vi "Display Data Queue manager.vi"(5 "queue size":i32, 7 "Action":T1=enum."Enqueue", 8 "error in":errorcluster, 11 "Data in":sgl[](array[numeric])) -> (0 "error out":errorcluster, 1 "# elements in queue":i32, 2 "Empty?":bool, 3 "data out":sgl[](array[numeric]))   [LabVIEW 2018]
uses:
  Controls/Queue Manager Actions.ctl
  Controls/QueueNames.ctl
  Controls/MessagePacket.ctl
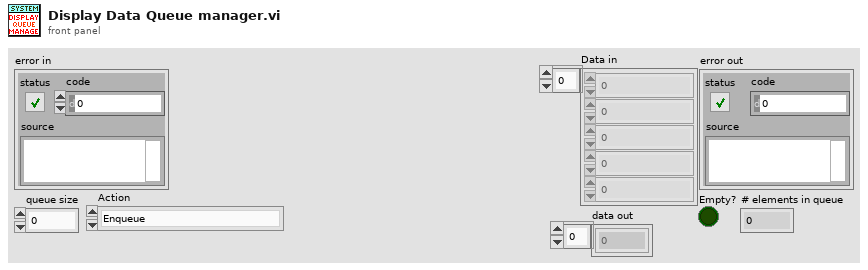
[diagram p1: front panel]
types:
  T1 = typedef "Queue Manager Actions.ctl" = enum16{"Init", "Enqueue", "Enqueue All", "Preview Queue", "Dequeue", "Get Status", "Flush Queue", "Flush All Queues", "Release All Queues", "Release Queue", "Enqueue at Opposite End"}
  T2 = typedef "MessagePacket.ctl" = cluster{"Message":string, "Parameter":variant}
  T3 = typedef "QueueNames.ctl" = enum16{"Main GUI", "Main Scan Processor", "Main Display Processing", "Main Processing", "Main Saving", "Main Display", "Main Table Stage GUI", "Main Table Stage Proc.", "Scan Engine", "Vibratome GUI", "Vibratome Processor", "Slice Engine"}
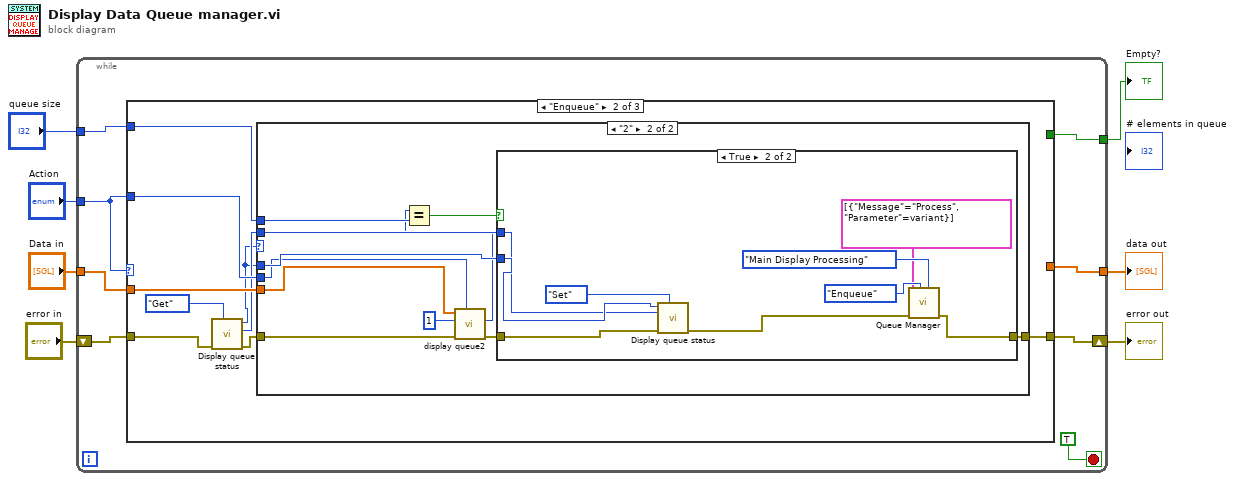
[diagram p0: block diagram]
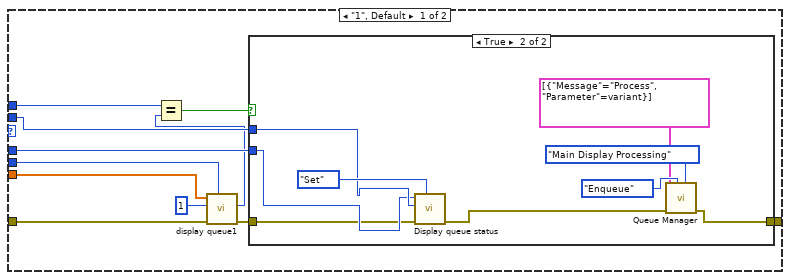
[diagram p3: hidden frame]
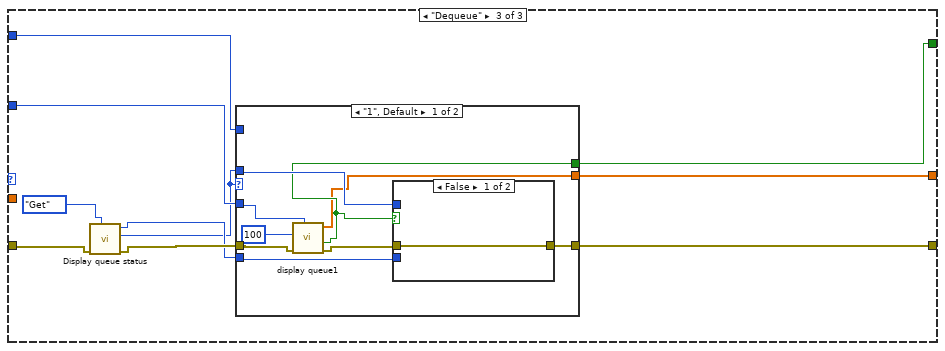
[diagram p6: hidden frame]
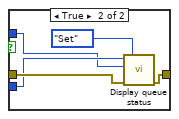
[diagram p7: hidden frame]
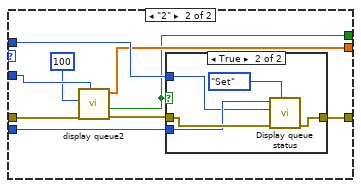
[diagram p8: hidden frame]
diagram:
  n1 = while {
    tunnel: "Data in" -> [w15]
    tunnel: "Action" -> [w14]
    tunnel: "queue size" -> [w12]
    shift-right: [w11] -> w3
    shift-left: "error in" -> [w13]
    tunnel: [w9] -> w2
    tunnel: [w8] -> w1
    stop <- TRUE stop-if-true
    n2 = case shown="\"Enqueue\"" w14 {
      tunnel: w15 -> [_ w25 _]
      tunnel: w13 -> [w16 w21 w72]
      tunnel: w14 -> [_ w24 w77]
      tunnel: w12 -> [_ w23 w76]
      tunnel: [w16 w22 w75] -> w11
      tunnel: [_ _ w74] -> w9
      tunnel: [_ _ w73] -> w8
      frame "Init", Default {
      }
      frame "Enqueue" {
        n3 = call "Display queue status.vi"("action"=enum16{"Init", "Get", "Set"}."Get", "error in"=w21) -> ("error out"=w17:errorcluster, "dequeue channel out"=w19:enum16{"1", "2"}, "enqueue channel out"=w18:enum16{"1", "2"})  [unwired: 6 in]
        n4 = case shown="\"2\"" w18 {
          tunnel: w25 -> [w31 w49]
          tunnel: w24 -> [w28 w51]
          tunnel: w17 -> [w27 w48]
          tunnel: w23 -> [w35 w57]
          tunnel: w18 -> [w33 w55]
          tunnel: w19 -> [w34 w54]
          tunnel: [w32 w53] -> w22
          frame "1", Default {
            n5 = call "display queue1.vi"("Action"=w28, "error in (no error)"=w27, "timeout in ms (-1)"=1, "data in"=w31) -> ("error out"=w29:errorcluster, "# elements in queue"=w26:i32)  [unwired: 4 in, 2 out]
            n6 = Equal?(x=w35, y=w26) -> (x = y?=w36:bool)
            n7 = case shown="True" w36 {
              tunnel: [w37 w40] -> w32
              tunnel: w29 -> [w37 w38]
              tunnel: w34 -> [_ w45]
              tunnel: w33 -> [_ w44]
              frame False {
              }
              frame True {
                n8 = call "Display queue status.vi"("action"=enum16{"Init", "Get", "Set"}."Set", "error in"=w38, "enqueue channel in"=w45, "dequeue channel in"=w44) -> ("error out"=w39:errorcluster)  [unwired: 4 in, 2 out]
                n9 = call "Queue Manager.vi"("Queue Name"=QueueNames."Main Display Processing", "Action"=Queue_Manager_Actions."Enqueue", "Error In"=w39, "Message Packet Array"=T2[] [{"Message"="Process", "Parameter"=variant}]) -> ("Error Out"=w40:errorcluster)  [unwired: 3 in, 4 out]
              }
            }
          }
          frame "2" {
            n10 = call "display queue2.vi"("Action"=w51, "error in (no error)"=w48, "timeout in ms (-1)"=1, "data in"=w49) -> ("error out"=w52:errorcluster, "# elements in queue"=w47:i32)  [unwired: 4 in, 2 out]
            n11 = Equal?(x=w47, y=w57) -> (x = y?=w56:bool)
            n12 = case shown="True" w56 {
              tunnel: w52 -> [w58 w60]
              tunnel: w55 -> [_ w66]
              tunnel: w54 -> [_ w65]
              tunnel: [w58 w61] -> w53
              frame False {
              }
              frame True {
                n13 = call "Display queue status.vi"("action"=enum16{"Init", "Get", "Set"}."Set", "error in"=w60, "enqueue channel in"=w65, "dequeue channel in"=w66) -> ("error out"=w59:errorcluster)  [unwired: 4 in, 2 out]
                n14 = call "Queue Manager.vi"("Queue Name"=QueueNames."Main Display Processing", "Action"=Queue_Manager_Actions."Enqueue", "Error In"=w59, "Message Packet Array"=T2[] [{"Message"="Process", "Parameter"=variant}]) -> ("Error Out"=w61:errorcluster)  [unwired: 3 in, 4 out]
              }
            }
          }
        }
      }
      frame "Dequeue" {
        n15 = call "Display queue status.vi"("action"=enum16{"Init", "Get", "Set"}."Get", "error in"=w72) -> ("error out"=w71:errorcluster, "dequeue channel out"=w68:enum16{"1", "2"}, "enqueue channel out"=w69:enum16{"1", "2"})  [unwired: 6 in]
        n16 = case shown="\"1\", Default" w68 {
          tunnel: w77 -> [w80 w95]
          tunnel: w71 -> [w83 w98]
          tunnel: w76 -> [_ _]
          tunnel: w69 -> [w85 w101]
          tunnel: w68 -> [w86 w100]
          tunnel: [w84 w99] -> w75
          tunnel: [w79 w93] -> w74
          tunnel: [w78 w96] -> w73
          frame "1", Default {
            n17 = call "display queue1.vi"("Action"=w80, "error in (no error)"=w83, "timeout in ms (-1)"=100) -> ("error out"=w82:errorcluster, "Empty?"=w79:bool, "data out"=w78:sgl[])  [unwired: 5 in, 1 out]
            n18 = case shown="False" w79 {
              tunnel: [w87 w91] -> w84
              tunnel: w82 -> [w87 w92]
              tunnel: w86 -> [_ w88]
              tunnel: w85 -> [_ w89]
              frame False {
              }
              frame True {
                n19 = call "Display queue status.vi"("action"=enum16{"Init", "Get", "Set"}."Set", "error in"=w92, "enqueue channel in"=w88, "dequeue channel in"=w89) -> ("error out"=w91:errorcluster)  [unwired: 4 in, 2 out]
              }
            }
          }
          frame "2" {
            n20 = call "display queue2.vi"("Action"=w95, "error in (no error)"=w98, "timeout in ms (-1)"=100) -> ("error out"=w97:errorcluster, "Empty?"=w93:bool, "data out"=w96:sgl[])  [unwired: 5 in, 1 out]
            n21 = case shown="True" w93 {
              tunnel: w101 -> [_ w104]
              tunnel: w100 -> [_ w103]
              tunnel: w97 -> [w102 w107]
              tunnel: [w102 w106] -> w99
              frame False {
              }
              frame True {
                n22 = call "Display queue status.vi"("action"=enum16{"Init", "Get", "Set"}."Set", "error in"=w107, "enqueue channel in"=w103, "dequeue channel in"=w104) -> ("error out"=w106:errorcluster)  [unwired: 4 in, 2 out]
              }
            }
          }
        }
      }
    }
  }
  "error out" <- w3
  "Empty?" <- w2
  "data out" <- w1
